vi "result judge single.vi"(0 "abs?":bool, 1 "limitType":enum16{"上限", "下限"}(ring), 2 "test value":dbl, 3 "limit":dbl) -> (8 "result string":string, 9 "pointSpec":string)   [LabVIEW 2011]
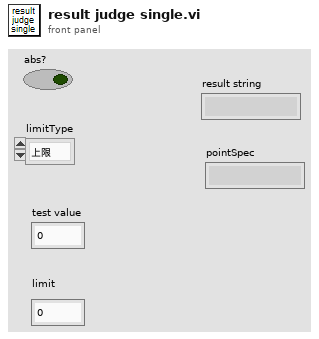
[diagram p1: front panel]
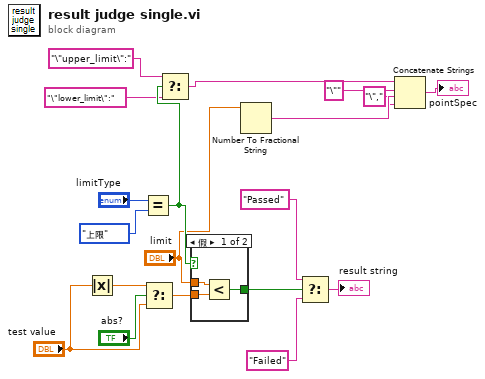
[diagram p0: block diagram]
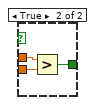
[diagram p2: hidden frame]
diagram:
  n1 = Absolute Value(x="test value") -> (abs(x)=w13:dbl)
  n2 = Equal?(x="limitType", y=enum16{"上限", "下限"}."上限" ("limit type")) -> (x = y?=w9:bool)
  n3 = Select(t=w13, s="abs?", f="test value") -> (s? t:f=w11:dbl)
  n4 = Select(t="\"upper_limit\":", s=w9, f="\"lower_limit\":") -> (s? t:f=w5:string)
  n5 = case shown="假" w9 {
    tunnel: "limit" -> [w22 w25]
    tunnel: w11 -> [w21 w24]
    tunnel: [w20 w23] -> w14
    frame False {
      n6 = Less?(x=w22, y=w21) -> (x < y?=w20:bool)
    }
    frame True {
      n7 = Greater?(x=w25, y=w24) -> (0:w23:bool)
    }
  }
  n8 = Number To Fractional String(number="limit") -> (F-format string=w4:string)  [unwired: 3 in]
  n9 = Select(t="Passed" ("TrueValue"), s=w14, f="Failed" ("FalseValue")) -> (s? t:f=→"result string":string)
  n10 = Concatenate Strings(w5, "\"" ("字符串"), w4, "\"," ("字符串")) -> (→"pointSpec":string)
